vi "Move South.vi"(11 "Map In":string[][](array[string])) -> (0 "Moved?":bool, 3 "Map Out":string[][](array[string]))   [LabVIEW 2021]
uses:
  <userlib>/_OpenG.lib/array/array.llb/Search 1D Array (String)__ogtk.vi
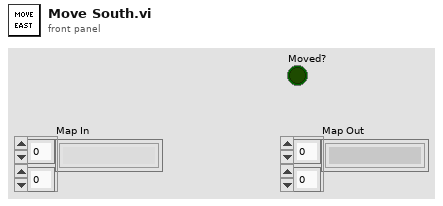
[diagram p1: front panel]
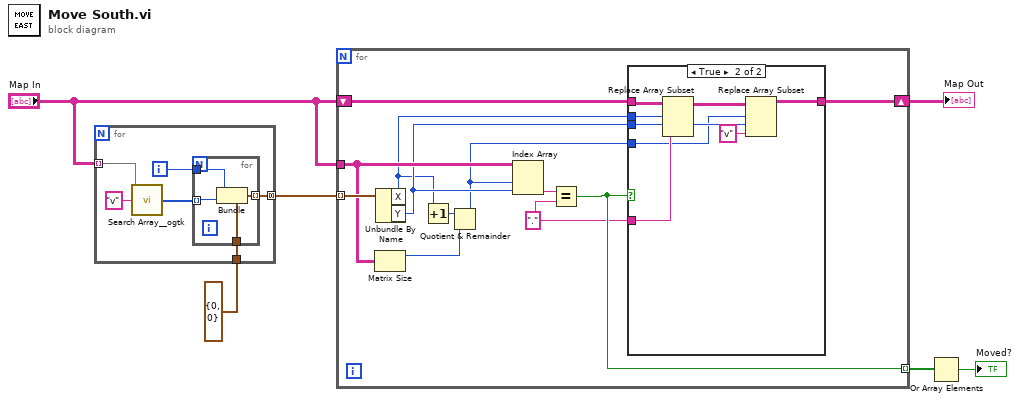
[diagram p0: block diagram]
diagram:
  n1 = for {
    tunnel: "Map In" -> [w12] mode=indexing
    tunnel: [w8] -> w5 mode=concatenating
    tunnel: cluster{"X":i32, "Y":i32} {"X"=0, "Y"=0} ("input cluster") -> [w7]
    i -> [w9]
    n2 = call-poly <userlib>:"Search Array__ogtk.vi"("Array"=w12, "Element Data"="v") -> ("Indices of Elements"=w10:i32[])  [unwired: 7 in]
    n3 = for {
      tunnel: w10 -> [w16] mode=indexing
      tunnel: w9 -> [w15]
      tunnel: [w14] -> w8 mode=indexing
      tunnel: w7 -> [w13]
      n4 = Bundle(cluster=w13, "X"=w15, "Y"=w16) -> (w14:cluster{"X":i32, "Y":i32})
    }
  }
  n5 = for {
    shift-right: [w23] -> w1
    shift-left: "Map In" -> [w24]
    tunnel: "Map In" -> [w26]
    tunnel: w5 -> [w28] mode=indexing
    tunnel: [w22] -> w3 mode=indexing
    w21 = "."
    n6 = Matrix Size(0:w26) -> (1:w18:i32)  [unwired: 1 out]
    n7 = Unbundle By Name(w28) -> ("X"=w19:i32, "Y"=w20:i32)
    n8 = Increment(x=w19) -> (x+1=w27:i32)
    n9 = Quotient & Remainder(x=w27, y=w18) -> (x-y*floor(x/y)=w17:i32)  [unwired: 1 out]
    n10 = Index Array(array=w26, index (row)=w17, index (col)=w20) -> (element=w25:string)
    n11 = Equal?(x=w25, y=w21) -> (x = y?=w22:bool)
    n12 = case shown="True" w22 {
      tunnel: w24 -> [w29 w37]
      tunnel: [w29 w35] -> w23
      tunnel: w19 -> [_ w34]
      tunnel: w20 -> [_ w31]
      tunnel: w21 -> [_ w33]
      tunnel: w17 -> [_ w30]
      frame False {
      }
      frame True {
        n13 = Replace Array Subset(array=w37, new element=w33, index (row)=w34, index (col)=w31) -> (w36:string[][])
        n14 = Replace Array Subset(array=w36, new element="v" ("new element/subarray"), index (row)=w30, index (col)=w31) -> (w35:string[][])
      }
    }
  }
  "Map Out" <- w1
  n15 = Or Array Elements(Boolean array=w3) -> (logical OR=→"Moved?":bool)
